vi "Read Device Identification.vi"(7 "unit ID":u8, 8 "error in":errorcluster, 9 "read device ID code":T2, 10 "object ID":u8, 11 "Modbus master in":refnum<class "Modbus Master.lvclass">) -> (0 "error out":errorcluster, 2 "objects":T1[](array[typedef]) {"Object ID" format="%x"}, 3 "Modbus master out":refnum<class "Modbus Master.lvclass">)   [LabVIEW 2013, in "Modbus Library - Advance.lvlib" / "Modbus Master.lvclass"]
doc: "Reads Modbus object information stored on the device. This can include basic information, like manufacturer, additional standard items, or model-specific extended items. This function may take a large amount of time to execute, as it requires the transfer of a large quantity of binary data. Even on TCP/IP, this function is limited by the maximum defined size of a Modbus protocol data unit."
uses:
  Modbus Master.lvclass
  Master Function Definition/Read Device ID code.ctl
  Data Model/Identification Parameters.ctl
  Modbus Master.lvclass/Modbus Master.ctl
  Modbus API.lvclass/Modbus API.ctl
  Transmission Data Unit/Transmission Data Unit.lvclass/Transmission Data Unit.ctl
  Transmission Data Unit/Transmission Data Unit.lvclass
  Data Model/Device Data Model.lvclass
  Modbus API.lvclass
  Master Function Definition/Master Function Definition.lvclass
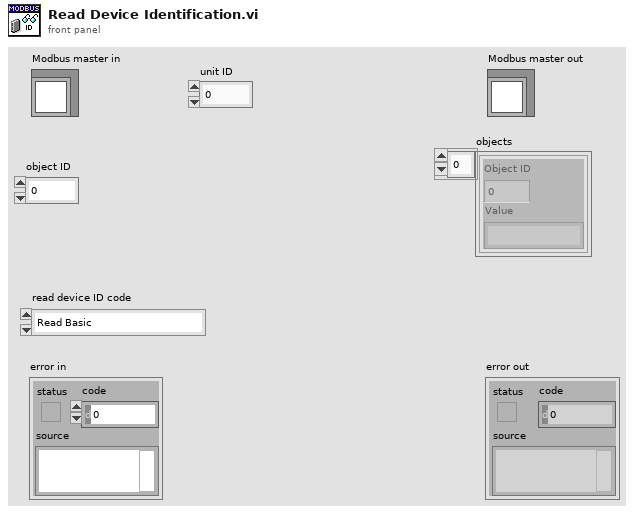
[diagram p1: front panel]
types:
  T1 = typedef "Modbus Library - Advance.lvlib/Device Data Model.lvclass/Identification Parameters.ctl" = cluster{"Object ID":u8, "Value":string}
  T2 = typedef "Modbus Library - Advance.lvlib/Device Data Model.lvclass/Read Device ID code.ctl" = enum8{"Read Basic", "Read Regular", "Read Extended", "Read Specific"}
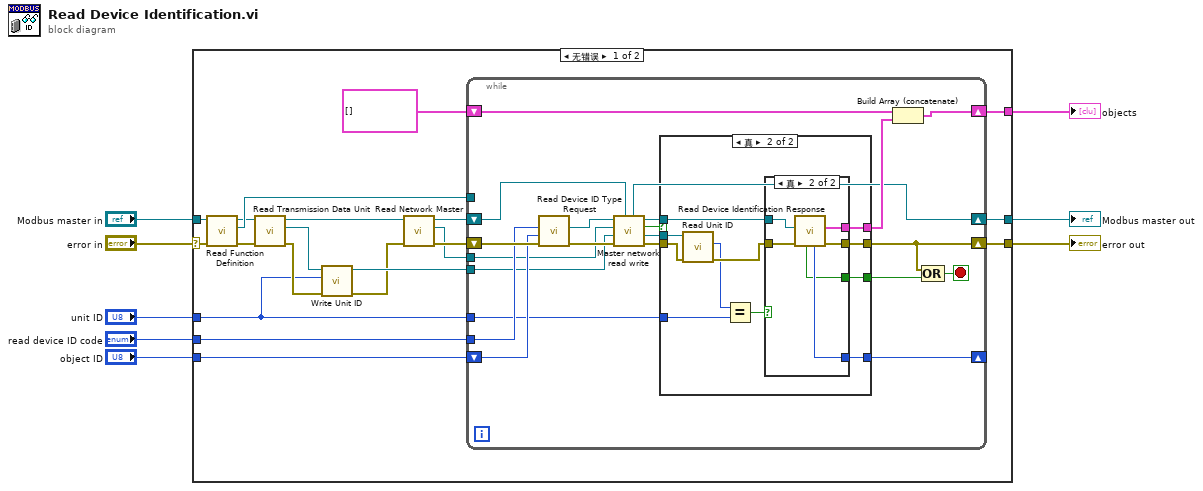
[diagram p0: block diagram]
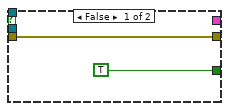
[diagram p2: hidden frame]
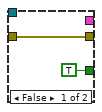
[diagram p3: hidden frame]
diagram:
  n1 = case shown="无错误" "error in" {
    selector: "error in" -> [w24 w72]
    tunnel: "Modbus master in" -> [w23 w71]
    tunnel: [w21 w71] -> w6
    tunnel: [w22 w72] -> w5
    tunnel: "read device ID code" -> [w28 _]
    tunnel: "object ID" -> [w27 _]
    tunnel: [w26 _] -> w2
    tunnel: "unit ID" -> [w9 _]
    frame No Error {
      n2 = call "Read Function Definition.vi"("error in"=w24, "Modbus master in"=w23) -> ("error out"=w16:errorcluster, "master function definition"=w20:refnum<class "Master Function Definition.lvclass">, "Modbus master out"=w15:refnum<class "Modbus Master.lvclass">)  [unwired: 7 in]
      n3 = call "Read Transmission Data Unit.vi"("error in"=w16, "Modbus instance in"=w15) -> ("error out"=w12:errorcluster, "transmission data unit"=w13:refnum<class "Transmission Data Unit.lvclass">, "Modbus instance out"=w17:refnum<class "Modbus Master.lvclass">)  [unwired: 7 in]
      n4 = call "Write Unit ID.vi"("error in"=w12, "unit ID"=w9, "transmission data unit in"=w13) -> ("error out"=w10:errorcluster, "transmission data unit out"=w11:refnum<class "Transmission Data Unit.lvclass">)  [unwired: 7 in]
      n5 = call "Read Network Master.vi"("error in"=w10, "Modbus master in"=w17) -> ("error out"=w19:errorcluster, "network master"=w14:refnum<class "Network Master.lvclass">, "Modbus master out"=w18:refnum<class "Modbus Master.lvclass">)  [unwired: 7 in]
      n6 = while {
        tunnel: w28 -> [w48]
        shift-right: [w45] -> w22
        shift-left: w19 -> [w49]
        shift-right: [w44] -> w26
        shift-left: T1[] [] -> [w43]
        shift-right: [w42] -> _
        shift-left: w27 -> [w47]
        shift-right: [w35] -> w21
        shift-left: w18 -> [w34]
        tunnel: w20 -> [_]
        tunnel: w11 -> [w33]
        tunnel: w14 -> [w32]
        tunnel: w9 -> [w30]
        stop <- w46 stop-if-true
        n7 = call "Read Device ID Type Request.vi"("error in"=w49, "Object ID"=w47, "Read Device ID Code"=w48) -> ("error out"=w36:errorcluster, "modbus data unit out"=w37:refnum<class "Modbus Data Unit.lvclass">)  [unwired: 7 in]
        n8 = call "Master network read write.vi"("Modbus master in"=w34, "error in"=w36, "transmission data unit in"=w33, "network master in"=w32, "Modbus data unit in"=w37) -> ("error out"=w39:errorcluster, "transmission data unit out"=w29:refnum<class "Transmission Data Unit.lvclass">, "PDU Valid?"=w31:bool, "Modbus data unit out"=w38:refnum<class "Modbus Data Unit.lvclass">, "Modbus master out"=w35:refnum<class "Modbus Master.lvclass">)  [unwired: 2 in]
        n9 = case shown="真" w31 {
          tunnel: [w51 w62] -> w45
          tunnel: [_ w61] -> w42
          tunnel: [TRUE ("done?") w60] -> w41
          tunnel: [_ w59] -> w40
          tunnel: w39 -> [w51 w56]
          tunnel: w38 -> [_ w58]
          tunnel: w30 -> [_ w53]
          tunnel: w29 -> [_ w57]
          frame False {
          }
          frame True {
            n10 = call "Read Unit ID.vi"("error in"=w56, "transmission data unit in"=w57) -> ("error out"=w55:errorcluster, "unit ID"=w54:u8)  [unwired: 7 in, 1 out]
            n11 = Equal?(x=w54, y=w53) -> (x = y?=w52:bool)
            n12 = case shown="真" w52 {
              tunnel: [w64 w70] -> w62
              tunnel: [_ w69] -> w61
              tunnel: [TRUE ("done?") w68] -> w60
              tunnel: [_ w67] -> w59
              tunnel: w58 -> [_ w66]
              tunnel: w55 -> [w64 w65]
              frame False {
              }
              frame True {
                n13 = call "Read Device Identification Response.vi"("error in"=w65, "modbus data unit in"=w66) -> ("error out"=w70:errorcluster, "Objects"=w67:T1[], "Next Object ID"=w69:u8, "done?"=w68:bool)  [unwired: 5 in, 1 out]
              }
            }
          }
        }
        n14 = Build Array (concatenate)(w43, w40) -> (w44:T1[])
        n15 = Compound Arithmetic op=OR(w45, w41) -> (w46:bool)
      }
    }
    frame Error {
    }
  }
  "error out" <- w5
  "Modbus master out" <- w6
  "objects" <- w2
